vi "ClearLastError.vi"(8 "error in (no error)":errorcluster, 11 "session id in":i32) -> (0 "error out":errorcluster, 3 "session id out":i32)   [LabVIEW 2017, in "libonnx_wrapper.lvlib"]
doc: "/**\n * @brief Очистить сообщение об ошибке для сессии\n * \n * Сбрасывает сохраненное сообщение об ошибке. Полезно после обработки ошибки,\n * чтобы не получить старое сообщение при следующей проверке.\n * \n * @param sessionId [IN] ID сессии\n * \n * @return void\n */\nvoid ClearLastError(int sessionId);"
uses:
  libonnx_wrapper.lvlib
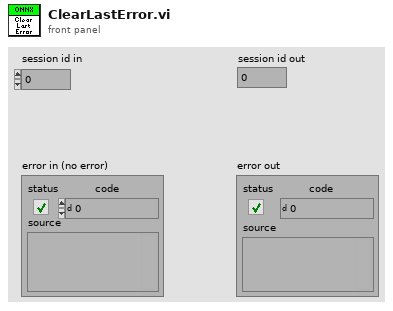
[diagram p1: front panel]
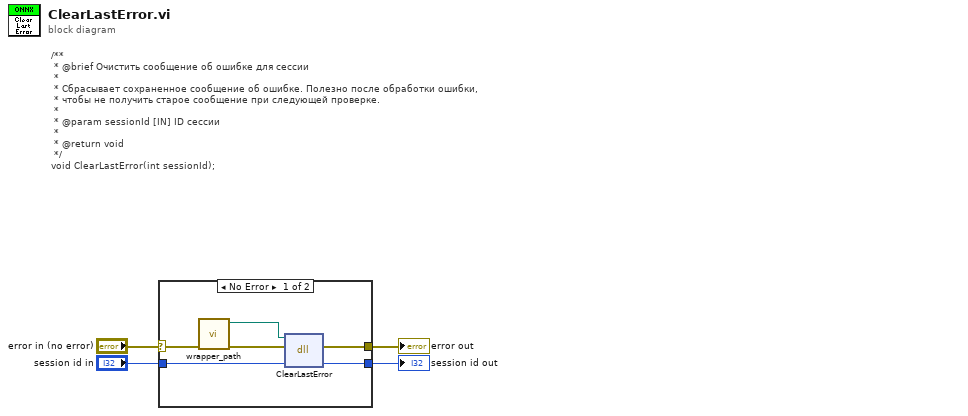
[diagram p0: block diagram]
diagram:
  # "/**\n * @brief Очистить сообщение об ошибке для сессии\n * \n * Сбрасывает сохраненное сообщение об ошибке. Полезно после обработки ошибки,\n * чтобы не получить старое сообщение при следующей проверке.\n * \n * @param sessionId [IN] ID сессии\n * \n * @return void\n */\nvoid ClearLastError(int sessionId);"
  n1 = case shown="No Error" "error in (no error)" {
    selector: "error in (no error)" -> [w5 w12]
    tunnel: [w10 w12] -> w4
    tunnel: "session id in" -> [w7 w11]
    tunnel: [w6 w11] -> w2
    frame No Error {
      n2 = call "wrapper_path.vi"("error in (no error)"=w5) -> ("error out"=w9:errorcluster, "wrapper path"=w8:path)  [unwired: 9 in]
      n3 = dll-call lib="home/ivan/LabVIEWData/ONNX/Test/libonnx_wrapper/unix64/libonnx_wrapper.so" fn="ClearLastError"(path in=w8, error in=w9, "sessionId"=w7) -> (error out=w10:errorcluster, "sessionId"=w6:i32)  [unwired: 2 in, 1 out]
    }
    frame Error {
    }
  }
  "error out" <- w4
  "session id out" <- w2
